vi "Choose Drive Command.vi"() -> (0 "Current Drive Command":T1)   [LabVIEW 2019]
uses:
  Drive Command Typedef.ctl
  Drive Mode Typedef.ctl
  .Team Code/Robot Global Data.vi
  Drive Global.vi
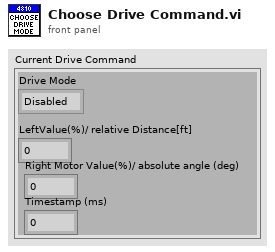
[diagram p1: front panel]
types:
  T1 = typedef "Drive Command Typedef.ctl" = cluster{"Drive Mode":T2, "LeftValue(%)/ relative Distance[ft]":dbl, "Right Motor Value(%)/ absolute angle (deg)":dbl, "Timestamp (ms)":dbl}
  T2 = typedef "Drive Mode Typedef.ctl" = enum16{"Disabled", "Auto-align", "Drive Distance", "Turn to angle", "Driver"}
  T3 = typedef "WPI_DriverStationRobotMode2.ctl" = enum16{"Autonomous Disabled", "Autonomous Enabled", "Teleop Disabled", "Teleop Enabled", "Disconnected", "Finish", "Test Disabled", "Test Enabled", "Emergency Stopped"}
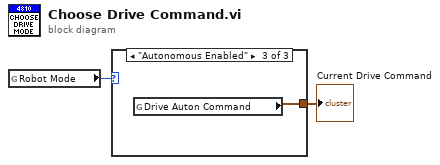
[diagram p0: block diagram]
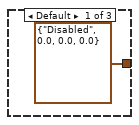
[diagram p2: hidden frame]
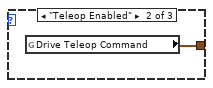
[diagram p3: hidden frame]
diagram:
  n1 = global read "Robot Global Data.vi" "Robot Mode"() -> (w2:T3)
  n2 = case shown="\"Autonomous Enabled\"" w2 {
    tunnel: [T1 {"Drive Mode"=enum."Disabled", "LeftValue(%)/ relative Distance[ft]"=0.0, "Right Motor Value(%)/ absolute angle (deg)"=0.0, "Timestamp (ms)"=0.0} ("Drive Command") w4 w5] -> w1
    frame Default {
    }
    frame "Teleop Enabled" {
      n3 = global read "Drive Global.vi" "Drive Teleop Command"() -> (w4:T1)
    }
    frame "Autonomous Enabled" {
      n4 = global read "Drive Global.vi" "Drive Auton Command"() -> (w5:T1)
    }
  }
  "Current Drive Command" <- w1
